vi "New Match.vi"(8 "error in (no error)":errorcluster, 9 "New Result Event":refnum<user-event>, 10 "GObj Refnum":refnum<vi>, 11 "Search in":refnum<class "Search.lvclass">) -> (0 "error out":errorcluster, 3 "Search out":refnum<class "Search.lvclass">)   [LabVIEW 2020, in "Better Search.lvlib" / "Search.lvclass"]
uses:
  Search.lvclass
  BetterSearch/Search Result.ctl
  Search Result/Search Result.lvclass
  Search.lvclass/Search.ctl
  Better Search.lvlib
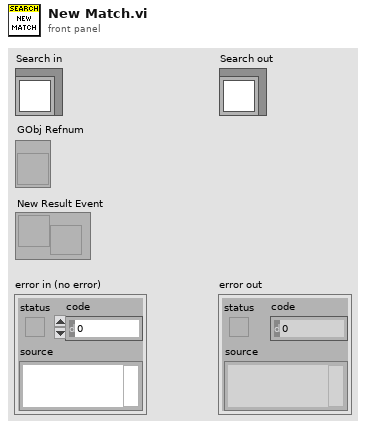
[diagram p1: front panel]
types:
  T1 = typedef "Better Search.lvlib/Search Result.ctl" = cluster{"Search":refnum<class "Search.lvclass">, "Result":refnum<class "Search Result.lvclass">}
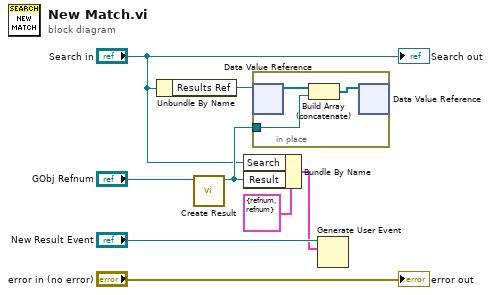
[diagram p0: block diagram]
diagram:
  n1 = Unbundle By Name("Search in") -> ("Results Ref"=w4:refnum<data-value>)
  n2 = call "Create Result.vi"("GObject"="GObj Refnum") -> ("Search Result out"=w3:refnum<class "Search Result.lvclass">)  [unwired: 9 in, 1 out]
  n3 = Bundle By Name(cluster=T1 {"Search"=refnum, "Result"=refnum} ("event data"), "Search"="Search in", "Result"=w3) -> (w5:T1)
  n4 = in-place {
    in-place-border: w3 -> [w10]
    n5 = in-place-dvr #1(w4) -> (w11:refnum<class "Search Result.lvclass">[])  [unwired: 1 out]
    n6 = Build Array (concatenate)(w11, w10) -> (w9:refnum<class "Search Result.lvclass">[])
    n7 = in-place-dvr #1(w9) -> ()  [unwired: 2 out]
  }
  n8 = Generate User Event(user event="New Result Event", event data cluster=w5) -> ()  [unwired: 2 in, 2 out]
  "error out" <- "error in (no error)"
  "Search out" <- "Search in"
